vi "Configure Gate.vi"(0 "VISA resource name":refnum<visa-resource-name>, 1 "Gate Signal Source (0:Wide IF Video)":i32(ring) items=["Wide IF Video", "External", "SG Marker", "Baseband Interface"], 2 "Gate Slope (0:Rise)":i32(ring) items=["Rise", "Fall"], 5 "Gate Sweep Delay (0ms)":dbl min=0.0 max=1000.0, 7 "Gate Length (20ms)":dbl=20.0 min=0.05 max=1000.0, 9 "Gate Level (-10.0dBm)":dbl=-10.0 min=-50.0 max=60.0 format="%.2f", 11 "error in (no error)":errorcluster, 12 "Gate Sweep Mode (0:Off)":i32(ring) items=["Off", "On"]) -> (4 "VISA resource name out":refnum<visa-resource-name>, 15 "error out":errorcluster)   [LabVIEW 2020, in "Anritsu Signal Analyzer Series.lvlib"]
doc: "Configures the gate settings of the spectrum analyzer."
uses:
  Anritsu Signal Analyzer Series.lvlib
panel:
  # "ms"
  # "ms"
  # "dBm"
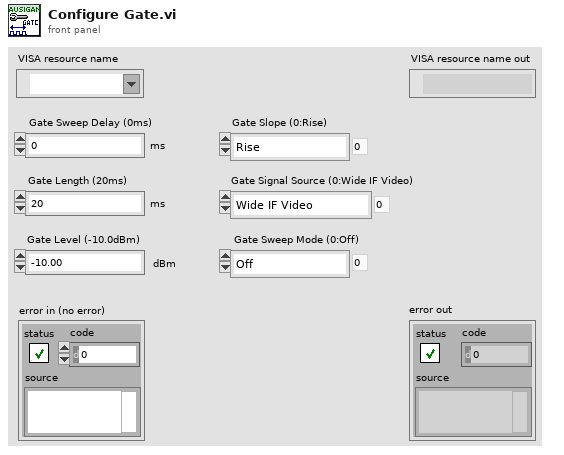
[diagram p1: front panel]
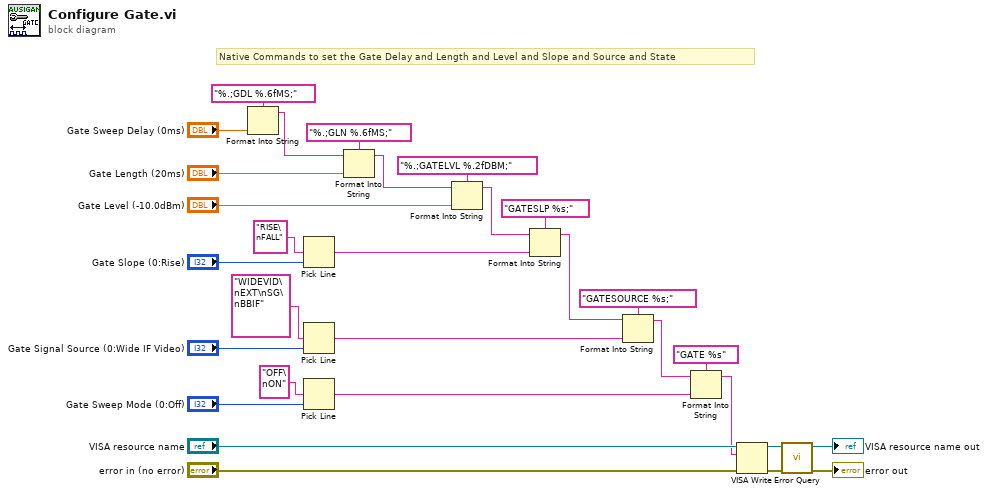
[diagram p0: block diagram]
diagram:
  # "Native Commands to set the Gate Delay and Length and Level and Slope and Source and State"
  n1 = Format Into String(format string="%.;GDL %.6fMS;" ("Format String"), "Gate Sweep Delay (0ms)") -> (resulting string=w16:string)  [unwired: 2 in, 1 out]
  n2 = Pick Line(multi-line string="RISE\nFALL" ("複数行文字列"), line index="Gate Slope (0:Rise)") -> (output string=w5:string)  [unwired: 1 in]
  n3 = Pick Line(multi-line string="WIDEVID\nEXT\nSG\nBBIF" ("複数行文字列"), line index="Gate Signal Source (0:Wide IF Video)") -> (output string=w3:string)  [unwired: 1 in]
  n4 = Pick Line(multi-line string="OFF\nON" ("複数行文字列"), line index="Gate Sweep Mode (0:Off)") -> (output string=w1:string)  [unwired: 1 in]
  n5 = Format Into String(format string="%.;GLN %.6fMS;" ("Format String"), initial string=w16, "Gate Length (20ms)") -> (resulting string=w14:string)  [unwired: 1 in, 1 out]
  n6 = Format Into String(format string="%.;GATELVL %.2fDBM;" ("Format String"), initial string=w14, "Gate Level (-10.0dBm)") -> (resulting string=w13:string)  [unwired: 1 in, 1 out]
  n7 = Format Into String(format string="GATESLP %s;" ("_CommandSet"), initial string=w13, w5) -> (resulting string=w11:string)  [unwired: 1 in, 1 out]
  n8 = Format Into String(format string="GATESOURCE %s;" ("_CommandSet"), initial string=w11, w3) -> (resulting string=w9:string)  [unwired: 1 in, 1 out]
  n9 = Format Into String(format string="GATE %s" ("_CommandSet"), initial string=w9, w1) -> (resulting string=w7:string)  [unwired: 1 in, 1 out]
  n10 = VISA Write(VISA resource name="VISA resource name", write buffer=w7, error in (no error)="error in (no error)") -> (VISA resource name out=w19:refnum<visa-resource-name>, error out=w18:errorcluster)  [unwired: 1 out]
  n11 = call "Error Query.vi"("error in (no error)"=w18, "VISA resource name"=w19) -> ("error out"=→"error out":errorcluster, "VISA resource name out"=→"VISA resource name out":refnum<visa-resource-name>)  [unwired: 6 in, 2 out]
